vi "LM model function and gradient (1-Exp, Convolved, Periodic, Fixed Parameters) v3.vi"(3 "output control":T1, 4 "data":variant, 5 "X":dbl[](array[numeric]), 6 "a (w sigma)":dbl[](array[numeric]) format="%_5g") -> (0 "error out":errorcluster, 1 "f'(X,a)":dbl[][](array[numeric]), 2 "f(X,a)":dbl[](array[numeric]))   [LabVIEW 2021, in "Fits.lvlib"]
doc: "This template is the starting point for creating a model function to be passed to the Nonlinear Curve Fit.vi."
uses:
  Fits.lvlib
  <vilib>/gmath/NumericalOptimization/LM_output select.ctl
  Fit Control Data v2.ctl
  Graphs/XY Graph/XY Plot Data.ctl
  IRF(X)PSED/Decay Fit Parameters In List.ctl
  Decay Model.ctl
  1-Exp Parameters.ctl
  Graphs/XY Graph/XY Graph Add-Ons.lvlib
  <vilib>/gmath/NI_Gmath.lvlib
panel:
  # "t0\n\nBL\n\nA1\n\nsqrt(tau1)"
  # "see the AlliGator License on the block diagram (Ctrl+E or Window:Show Block Diagram)"
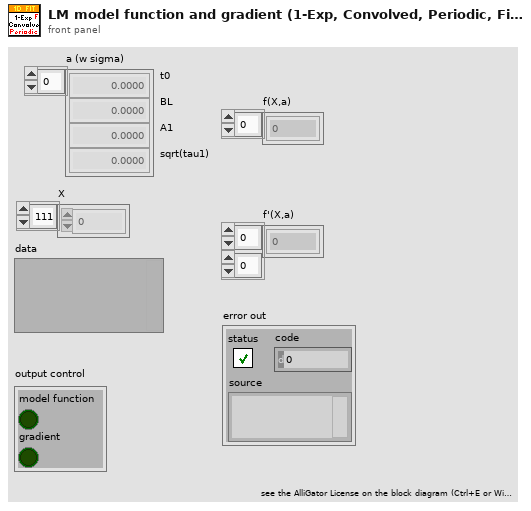
[diagram p1: front panel]
types:
  T1 = typedef "NI_Gmath.lvlib/LM_output select.ctl" = cluster{"model function":bool, "gradient":bool}
  T2 = typedef "Fits.lvlib/1-Exp Parameters.ctl" = cluster{"t_0":dbl, "B":dbl, "A":dbl, "tau":dbl, "T":dbl, "sigma":dbl}
  T3 = typedef "Fits.lvlib/Fit Control Data v2.ctl" = cluster{"IRF":T4, "Laser Period":dbl, "SYNC Period":dbl, "Fixed Parameter Names":T5[], "Fixed Parameter Values":dbl[], "Fitted Parameter Names":T5[], "Fit Model":T6}
  T4 = typedef "XY Graph Add-Ons.lvlib/XY Plot Data.ctl" = cluster{"X Array":dbl[], "Y Array":dbl[]}
  T5 = typedef "Fits.lvlib/Decay Fit Parameters In List.ctl" = enum16{"Offset", "Baseline", "A_1", "tau_1", "A_2", "tau_2"}
  T6 = typedef "Fits.lvlib/Decay Model.ctl" = enum16{"1-Exponential", "2-Exponentials"}
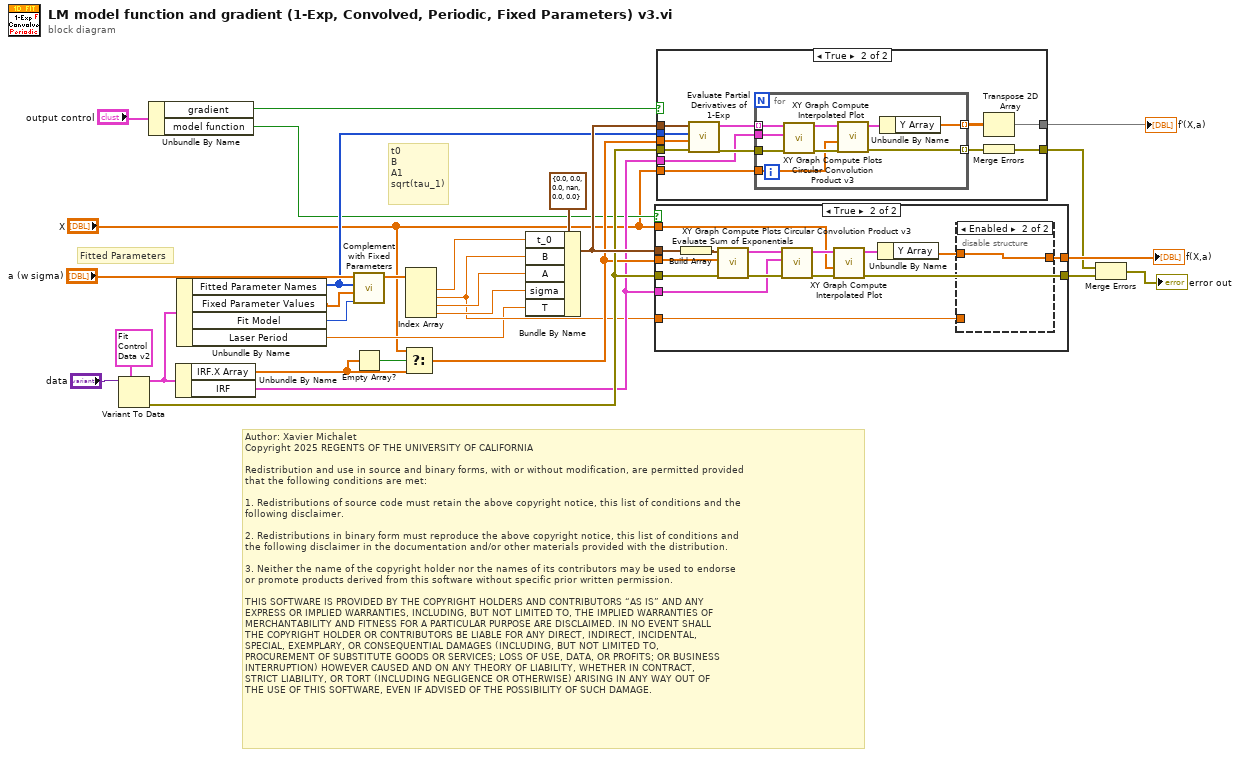
[diagram p0: block diagram]
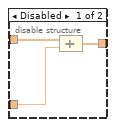
[diagram p3: hidden frame]
diagram:
  # "Author: Xavier Michalet\nCopyright 2025 REGENTS OF THE UNIVERSITY OF CALIFORNIA\n\nRedistribution and use in source and binary forms, with or without modification, are permitted provided\nthat the following conditions are met:\n\n1. Redistributions of source code must retain the above copyright notice, this list of conditions and the\nfollowing disclaimer.\n\n2. Redistributions in binary form must reproduce the above copyright notice, this list of conditions and\nthe following disclaimer in the documentation and/or other materials provided with the distribution.\n\n3. Neither the name of the copyright holder nor the names of its contributors may be used to endorse \nor promote products derived from this software without specific prior written permission.\n\nTHIS SOFTWARE IS PROVIDED BY THE COPYRIGHT HOLDERS AND CONTRIBUTORS “AS IS” AND ANY \nEXPRESS OR IMPLIED WARRANTIES, INCLUDING, BUT NOT LIMITED TO, THE IMPLIED WARRANTIES OF\nMERCHANTABILITY AND FITNESS FOR A PARTICULAR PURPOSE ARE DISCLAIMED. IN NO EVENT SHALL\nTHE COPYRIGHT HOLDER OR CONTRIBUTORS BE LIABLE FOR ANY DIRECT, INDIRECT, INCIDENTAL, \nSPECIAL, EXEMPLARY, OR CONSEQUENTIAL DAMAGES (INCLUDING, BUT NOT LIMITED TO, \nPROCUREMENT OF SUBSTITUTE GOODS OR SERVICES; LOSS OF USE, DATA, OR PROFITS; OR BUSINESS\nINTERRUPTION) HOWEVER CAUSED AND ON ANY THEORY OF LIABILITY, WHETHER IN CONTRACT, \nSTRICT LIABILITY, OR TORT (INCLUDING NEGLIGENCE OR OTHERWISE) ARISING IN ANY WAY OUT OF\nTHE USE OF THIS SOFTWARE, EVEN IF ADVISED OF THE POSSIBILITY OF SUCH DAMAGE."
  # "Fitted Parameters"
  # "t0\nB\nA1\nsqrt(tau_1)"
  n1 = Variant To Data(type=T3 {"IRF"={"X Array"=[], "Y Array"=[]}, "Laser Period"=0.0, "SYNC Period"=0.0, "Fixed Parameter Names"=[], "Fixed Parameter Values"=[], "Fitted Parameter Names"=[], "Fit Model"=enum."1-Exponential"} ("Fit Control Data"), Variant="data") -> (data=w21:T3, error out=w13:errorcluster)  [unwired: 1 in]
  n2 = Unbundle By Name("output control") -> ("gradient"=w10:bool, "model function"=w8:bool)
  n3 = Unbundle By Name(w21) -> ("IRF.X Array"=w1:dbl[], "IRF"=w9:T4)
  n4 = Unbundle By Name(w21) -> ("Fitted Parameter Names"=w14:T5[], "Fixed Parameter Values"=w18:dbl[], "Fit Model"=w17:T6, "Laser Period"=w4:dbl)
  n5 = call "Complement with Fixed Parameters.vi"("Fit Model"=w17, "Fixed Parameter Values"=w18, "Fitted Parameter Names"=w14, "a in"="a (w sigma)") -> ("a out"=w20:dbl[])  [unwired: 7 in]
  n6 = Empty Array?(array=w1) -> (empty?=w2:bool)
  n7 = Select(t="X", s=w2, f=w1) -> (s? t:f=w12:dbl[])
  n8 = Index Array(array=w20) -> (element #1=w24:dbl, element #2=w5:dbl, element #3=w23:dbl, element #4=w26:dbl)  [unwired: 4 in]
  n9 = Bundle By Name(cluster=T2 {"t_0"=0.0, "B"=0.0, "A"=0.0, "tau"=nan, "T"=0.0, "sigma"=0.0} ("Gate & Decay Parameters"), "t_0"=w24, "B"=w5, "A"=w23, "sigma"=w26, "T"=w4) -> (w15:T2)
  n10 = case shown="True" w8 {
    tunnel: [_ w45] -> w25
    tunnel: w5 -> [_ w41]
    tunnel: [w30 w37] -> w22
    tunnel: w15 -> [_ w36]
    tunnel: w13 -> [w30 w35]
    tunnel: w12 -> [_ w33]
    tunnel: "X" -> [_ w32]
    tunnel: w9 -> [_ w31]
    frame False {
    }
    frame True {
      n11 = Build Array(w36) -> (w44:T2[])
      n12 = call "Evaluate Sum of Exponentials.vi"("error in (no error)"=w35, "Ramp"=w33, "Exp Parameters Array"=w44) -> ("error out"=w42:errorcluster, "Plot"=w34:T4)  [unwired: 7 in]
      n13 = call "XY Graph Compute Plots Circular Convolution Product v3.vi"("Error In"=w42, "Plot 2 (kernel)"=w31, "Plot 1 (function)"=w34) -> ("Error Out"=w38:errorcluster, "Convolution Product"=w40:T4)  [unwired: 6 in, 1 out]
      n14 = call "XY Graph Compute Interpolated Plot.vi"("Error In"=w38, "Ramp"=w32, "Plot"=w40) -> ("Error Out"=w37:errorcluster, "Interpolated Plot"=w39:T4)  [unwired: 7 in]
      n15 = Unbundle By Name(w39) -> ("Y Array"=w43:dbl[])
      n16 = disable-structure shown="Enabled" {
        disable-tunnel: [w48 w49] -> w45
        disable-tunnel: w43 -> [w47 w49]
        disable-tunnel: w41 -> [w46 _]
        frame Disabled {
          n17 = Compound Arithmetic op=ADD(w47, w46) -> (w48:dbl[])
        }
        frame Enabled {
        }
      }
    }
  }
  "f(X,a)" <- w25
  n18 = case shown="True" w10 {
    tunnel: w15 -> [_ w62]
    tunnel: w14 -> [_ w61]
    tunnel: w13 -> [w50 w60]
    tunnel: w12 -> [_ w58]
    tunnel: [_ w55] -> w11
    tunnel: "X" -> [_ w54]
    tunnel: w9 -> [_ w53]
    tunnel: [w50 w51] -> w6
    frame False {
    }
    frame True {
      n19 = call "Evaluate Partial Derivatives of 1-Exp.vi"("error in (no error)"=w60, "Ramp"=w58, "Fitted Parameter Names"=w61, "Exp Parameters"=w62) -> ("error out"=w57:errorcluster, "Partial Derivatives Plot Array"=w59:T4[])  [unwired: 6 in]
      n20 = for {
        tunnel: w59 -> [w71] mode=indexing
        tunnel: w53 -> [w70]
        tunnel: w57 -> [w69]
        tunnel: w54 -> [w66]
        tunnel: [w64] -> w56 mode=indexing
        tunnel: [w63] -> w52 mode=indexing
        n21 = call "XY Graph Compute Plots Circular Convolution Product v3.vi"("Error In"=w69, "Plot 2 (kernel)"=w70, "Plot 1 (function)"=w71) -> ("Error Out"=w68:errorcluster, "Convolution Product"=w67:T4)  [unwired: 6 in, 1 out]
        n22 = call "XY Graph Compute Interpolated Plot.vi"("Error In"=w68, "Ramp"=w66, "Plot"=w67) -> ("Error Out"=w63:errorcluster, "Interpolated Plot"=w65:T4)  [unwired: 7 in]
        n23 = Unbundle By Name(w65) -> ("Y Array"=w64:dbl[])
      }
      n24 = Transpose 2D Array(2D array=w56) -> (transposed array=w55:dbl[][])
      n25 = Merge Errors(w52) -> (w51:errorcluster)
    }
  }
  "f'(X,a)" <- w11
  n26 = Merge Errors(w6, w22) -> (→"error out":errorcluster)
